vi "ShortcutMenu.vi"(8 "error in":errorcluster, 9 "menu ref in":refnum<k9>, 11 "node in":refnum<class "module editor node.lvclass">) -> (0 "error out":errorcluster, 1 "menu ref out":refnum<k9>, 3 "node out":refnum<class "module editor node.lvclass">)   [LabVIEW 2013, in "PL Framework Configuration Tool.lvlib" / "module editor node.lvclass"]
doc: "Defines the behavior of the shortcut menu of the node."
uses:
  module editor node.lvclass
  Allowed Execution Modes.ctl
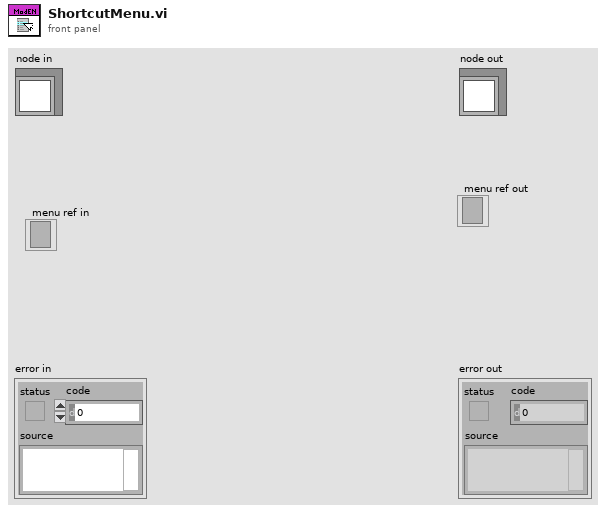
[diagram p1: front panel]
types:
  T1 = typedef "PL Framework Configuration Tool.lvlib/module editor node.lvclass/Allowed Execution Modes.ctl" = enum16{"Synchronous", "Asynchronous"}
  T2 = typedef "NISE_CEF_Node.lvclass/NodeMenuOptions.ctl" = cluster{"removable":bool, "movable":bool, "duplicate":bool}
  T3 = typedef "NISE_CEF_Node.lvclass/SubNodeCluster.ctl" = cluster{"subnodes menu name":string[], "subnodes class":string[]}
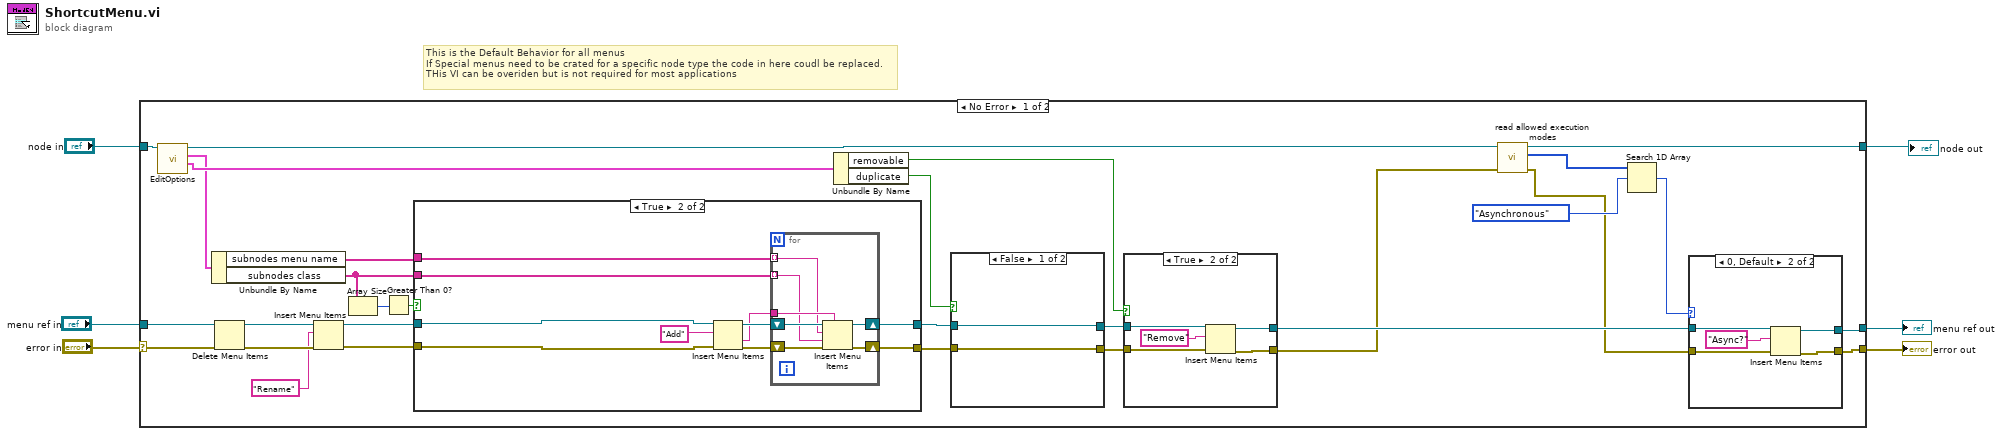
[diagram p0: block diagram]
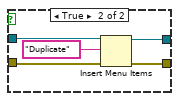
[diagram p4: hidden frame]
diagram:
  # "This is the Default Behavior for all menus\nIf Special menus need to be crated for a specific node type the code in here coudl be replaced.\nTHis VI can be overiden but is not required for most applications"
  n1 = case shown="No Error" "error in" {
    selector: "error in" -> [w27 w78]
    tunnel: [w19 w79] -> w4
    tunnel: "node in" -> [w30 w79]
    tunnel: "menu ref in" -> [w31 w77]
    tunnel: [w16 w78] -> w5
    tunnel: [w17 w77] -> w6
    frame No Error {
      n2 = call-dynamic "EditOptions.vi"("Module Editor Node in"=w30) -> ("edit options"=w29:T2, "subnodes class"=w23:T3, "Module Editor Node out"=w20:refnum<class "module editor node.lvclass">)  [unwired: 7 in, 1 out]
      n3 = Unbundle By Name(w23) -> ("subnodes menu name"=w22:string[], "subnodes class"=w21:string[])
      n4 = Delete Menu Items(6:w27, 9:w31) -> (0:w34:errorcluster, 3:w12:refnum<k9>)  [unwired: 2 in]
      n5 = Insert Menu Items(6:w34, 8:"Rename", 9:w12) -> (0:w13:errorcluster, 3:w11:refnum<k9>)  [unwired: 3 in, 1 out]
      n6 = Array Size(array=w21) -> (size(s)=w36:i32)
      n7 = Greater Than 0?(x=w36) -> (x > 0?=w35:bool)
      n8 = case shown="True" w35 {
        tunnel: w11 -> [w59 w60]
        tunnel: w13 -> [w58 w69]
        tunnel: w22 -> [_ w64]
        tunnel: [w59 w63] -> w33
        tunnel: [w58 w62] -> w32
        tunnel: w21 -> [_ w61]
        frame False {
        }
        frame True {
          n9 = Insert Menu Items(6:w69, 8:"Add", 9:w60) -> (0:w66:errorcluster, 1:w65:string, 3:w67:refnum<k9>)  [unwired: 3 in]
          n10 = for {
            tunnel: w65 -> [w74]
            tunnel: w64 -> [w71] mode=indexing
            shift-right: [w73] -> w63
            shift-left: w67 -> [w76]
            shift-right: [w72] -> w62
            shift-left: w66 -> [w75]
            tunnel: w61 -> [w70] mode=indexing
            n11 = Insert Menu Items(5:w74, 6:w75, 7:w70, 8:w71, 9:w76) -> (0:w72:errorcluster, 3:w73:refnum<k9>)  [unwired: 1 in, 1 out]
          }
        }
      }
      n12 = Unbundle By Name(w29) -> ("removable"=w24:bool, "duplicate"=w28:bool)
      n13 = case shown="False" w28 {
        tunnel: w33 -> [w52 w57]
        tunnel: w32 -> [w51 w56]
        tunnel: [w52 w55] -> w25
        tunnel: [w51 w54] -> w26
        frame False {
        }
        frame True {
          n14 = Insert Menu Items(6:w56, 8:"Duplicate", 9:w57) -> (0:w54:errorcluster, 3:w55:refnum<k9>)  [unwired: 3 in, 1 out]
        }
      }
      n15 = case shown="True" w24 {
        tunnel: w26 -> [w45 w50]
        tunnel: [w45 w49] -> w9
        tunnel: w25 -> [w44 w48]
        tunnel: [w44 w46] -> w18
        frame False {
        }
        frame True {
          n16 = Insert Menu Items(6:w50, 8:"Remove", 9:w48) -> (0:w49:errorcluster, 3:w46:refnum<k9>)  [unwired: 3 in, 1 out]
        }
      }
      n17 = call-dynamic "read allowed execution modes.vi"("error in"=w9, "Module Editor Node in"=w20) -> ("error out"=w7:errorcluster, "allowed execution modes"=w8:T1[], "Module Editor Node out"=w19:refnum<class "module editor node.lvclass">)  [unwired: 7 in]
      n18 = Search 1D Array(1D array=w8, element=Allowed_Execution_Modes."Asynchronous") -> (index of element=w14:i32)  [unwired: 1 in]
      n19 = case shown="0, Default" w14 {
        tunnel: w7 -> [w38 w43]
        tunnel: [w38 w42] -> w16
        tunnel: w18 -> [w37 w41]
        tunnel: [w37 w39] -> w17
        frame -1 {
        }
        frame 0, Default {
          n20 = Insert Menu Items(6:w43, 8:"Async?", 9:w41) -> (0:w42:errorcluster, 3:w39:refnum<k9>)  [unwired: 3 in, 1 out]
        }
      }
    }
    frame Error {
    }
  }
  "error out" <- w5
  "node out" <- w4
  "menu ref out" <- w6
